vi "create file.vi"(8 "error in (no error)":errorcluster, 11 "Log File in":refnum<class "CCS_Log File.lvclass">) -> (0 "error out":errorcluster, 3 "Log File out":refnum<class "CCS_Log File.lvclass">)   [LabVIEW 2018, in "CCS_Log File.lvclass"]
uses:
  CCS_Log File.lvclass
  CCS_Log File.lvclass/CCS_Log File.ctl
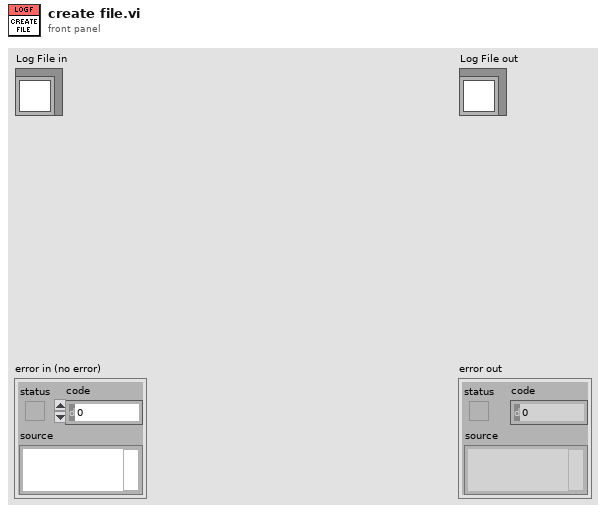
[diagram p1: front panel]
types:
  T1 = enum16{"open", "replace", "create", "open or create", "replace or create", "replace or create with confirmation"}
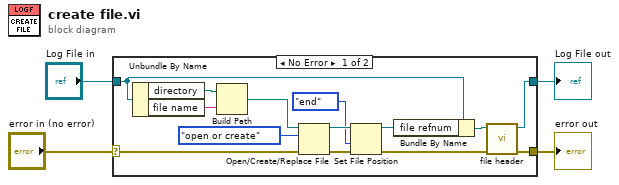
[diagram p0: block diagram]
diagram:
  n1 = case shown="No Error" "error in (no error)" {
    selector: "error in (no error)" -> [w18 w20]
    tunnel: [w11 w20] -> w3
    tunnel: [w12 w19] -> w1
    tunnel: "Log File in" -> [w15 w19]
    frame No Error {
      n2 = Unbundle By Name(w15) -> ("directory"=w10:path, "file name"=w17:string)
      n3 = Build Path(base path=w10, name or relative path=w17) -> (appended path=w16:path)
      n4 = Open/Create/Replace File(file path (use dialog)=w16, error in=w18, operation (0:open)=T1."open or create") -> (refnum out=w6:refnum<file>, error out=w9:errorcluster)  [unwired: 3 in, 1 out]
      n5 = Set File Position(refnum=w6, from (0:start)=enum16{"start", "end", "current"}."end", error in=w9) -> (refnum out=w7:refnum<file>, error out=w8:errorcluster)  [unwired: 1 in]
      n6 = Bundle By Name(cluster=w15, "file refnum"=w7) -> (w13:refnum<class "CCS_Log File.lvclass">)
      n7 = call-dynamic "file header.vi"("error in (no error)"=w8, "Log File in"=w13) -> ("error out"=w11:errorcluster, "Log File out"=w12:refnum<class "CCS_Log File.lvclass">)  [unwired: 8 in]
    }
    frame Error {
    }
  }
  "error out" <- w3
  "Log File out" <- w1
